vi "Save Notebook Rich Text Box.vi"(6 "Backup?":bool, 7 "Default Notebook File Name (Notebook)":string="Notebook", 8 "Error In":errorcluster, 9 "Dialog (F)":bool, 10 "File Path Control":path, 11 ".NET Refnum in":refnum<k24>) -> (0 "Error Out":errorcluster, 1 "cancelled":bool, 2 "File Path out":path, 3 "Rtf Content":string)   [LabVIEW 2021, in "Notebook.lvlib"]
uses:
  Notebook.lvlib
  System.Windows.Forms
  Rich Text Box/Text Format List.ctl
  GUI/GUI.lvlib
  Files/Files.lvlib
  Rich Text Box/Rich Text Box.lvlib
  Strings/Strings.lvlib
panel:
  # "see the License on the block diagram (Ctrl+E or Window:Show Block Diagram)"
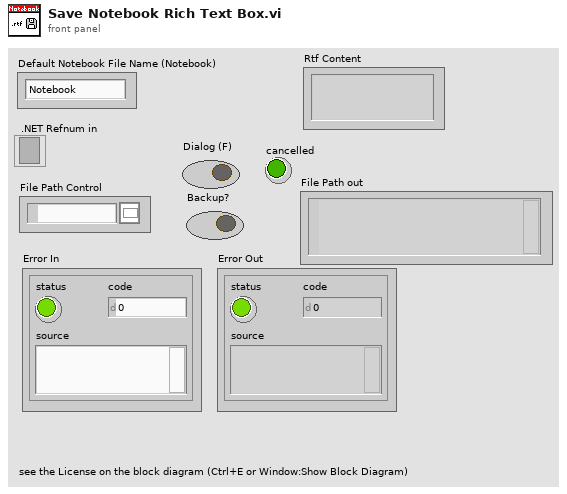
[diagram p1: front panel]
types:
  T1 = typedef "Notebook.lvlib/Text Format List.ctl" = enum16{"Message", "Result", "Error", "Setting", "Verbose", "Warning"}
  T2 = typedef "Rich Text Box.lvlib/Text Formatting.ctl" = cluster{"Font":string, "Text Color":T3, "Background Color":T3, "Style":T4, "Font Size":dbl, "Alignment":T5}
  T3 = typedef "Rich Text Box.lvlib/Text Colors.ctl" = enum16{"Unchanged", "Black", "Blue", "Cyan", "Maroon", "Gray", "Violet", "Green", "Light Green", "Orange", "Yellow", "Magenta", "Red", "White"}
  T4 = typedef "Rich Text Box.lvlib/Text Style.ctl" = enum16{"Regular", "Bold", "Italic", "Underline", "Strikeout"}
  T5 = typedef "Rich Text Box.lvlib/Text Alignment.ctl" = enum16{"Left", "Right", "Center"}
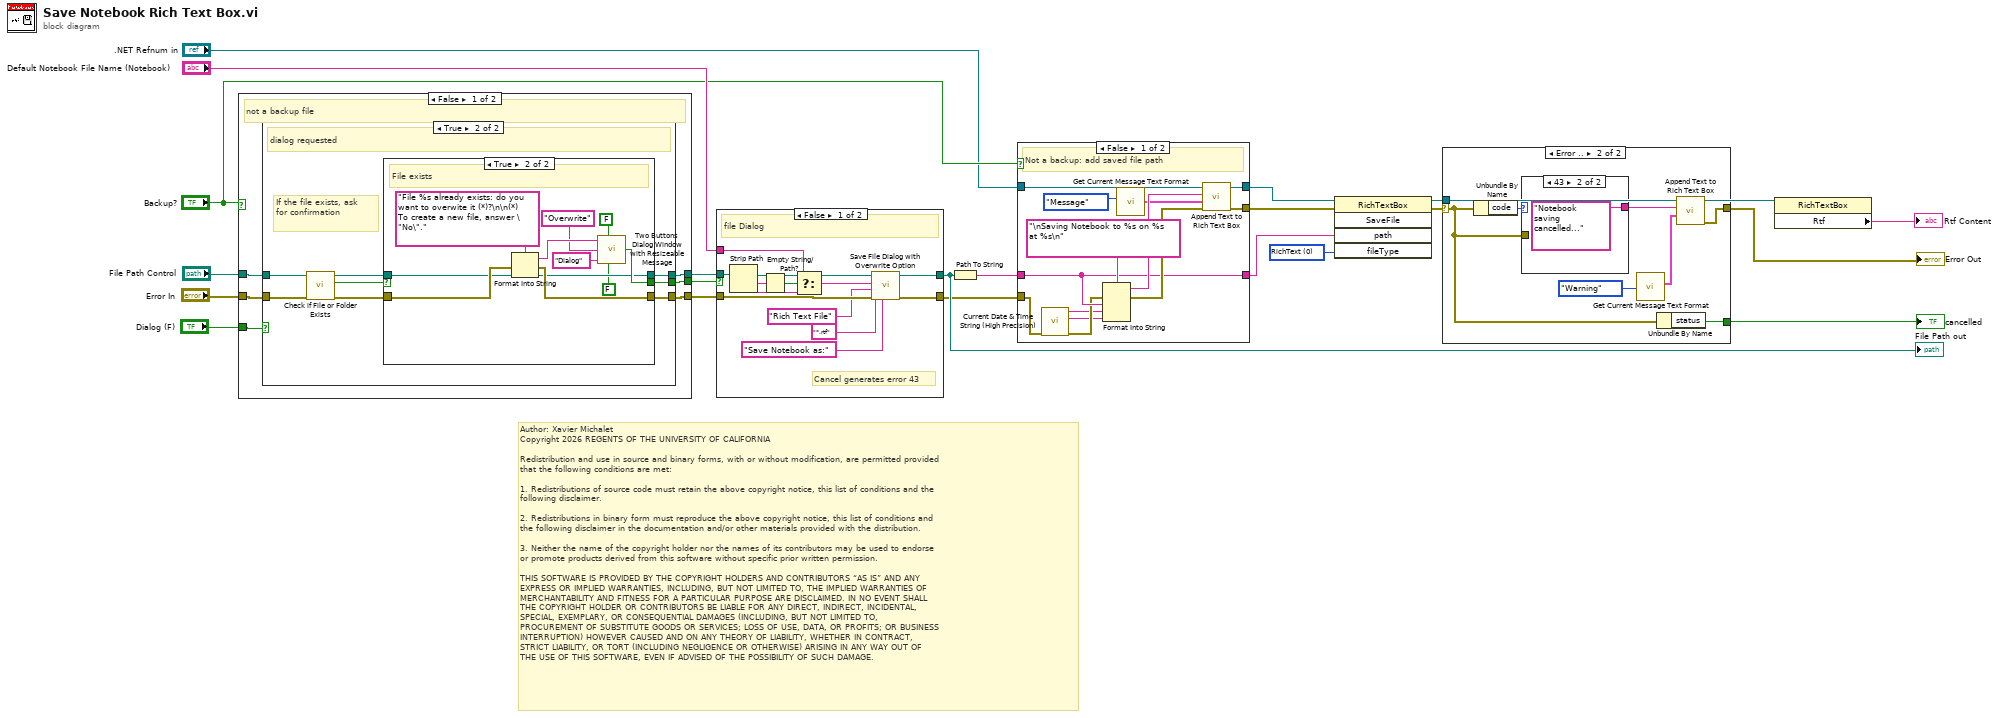
[diagram p0: block diagram]
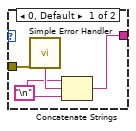
[diagram p4: hidden frame]
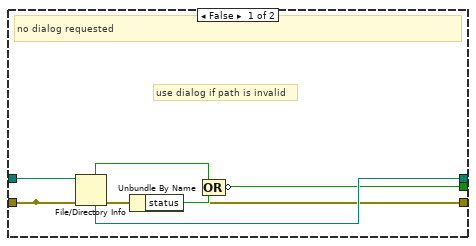
[diagram p6: hidden frame]
diagram:
  w20 = 0 items=["RichText", "PlainText", "RichNoOleObjs", "TextTextOleObjs", "UnicodePlainText"] ("fileType")
  # "Author: Xavier Michalet\nCopyright 2026 REGENTS OF THE UNIVERSITY OF CALIFORNIA\n\nRedistribution and use in source and binary forms, with or without modification, are permitted provided\nthat the following conditions are met:\n\n1. Redistributions of source code must retain the above copyright notice, this list of conditions and the\nfollowing disclaimer.\n\n2. Redistributions in binary form must reproduce the above copyright notice, this list of conditions and\nthe following disclaimer in the documentation and/or other materials provided with the distribution.\n\n3. Neither the name of the copyright holder nor the names of its contributors may be used to endorse \nor promote products derived from this software without specific prior written permission.\n\nTHIS SOFTWARE IS PROVIDED BY THE COPYRIGHT HOLDERS AND CONTRIBUTORS “AS IS” AND ANY \nEXPRESS OR IMPLIED WARRANTIES, INCLUDING, BUT NOT LIMITED TO, THE IMPLIED WARRANTIES OF\nMERCHANTABILITY AND FITNESS FOR A PARTICULAR PURPOSE ARE DISCLAIMED. IN NO EVENT SHALL\nTHE COPYRIGHT HOLDER OR CONTRIBUTORS BE LIABLE FOR ANY DIRECT, INDIRECT, INCIDENTAL, \nSPECIAL, EXEMPLARY, OR CONSEQUENTIAL DAMAGES (INCLUDING, BUT NOT LIMITED TO, \nPROCUREMENT OF SUBSTITUTE GOODS OR SERVICES; LOSS OF USE, DATA, OR PROFITS; OR BUSINESS\nINTERRUPTION) HOWEVER CAUSED AND ON ANY THEORY OF LIABILITY, WHETHER IN CONTRACT, \nSTRICT LIABILITY, OR TORT (INCLUDING NEGLIGENCE OR OTHERWISE) ARISING IN ANY WAY OUT OF\nTHE USE OF THIS SOFTWARE, EVEN IF ADVISED OF THE POSSIBILITY OF SUCH DAMAGE."
  n1 = case shown="False" "Backup?" {
    selector: "Backup?" -> [_ w58]
    tunnel: [w25 w57] -> w19
    tunnel: [w27 w56] -> w18
    tunnel: [w26 w58] -> w17
    tunnel: "Dialog (F)" -> [w22 _]
    tunnel: "File Path Control" -> [w24 w57]
    tunnel: "Error In" -> [w23 w56]
    frame False {
      # "not a backup file"
      n2 = case shown="True" w22 {
        tunnel: [w28 w42] -> w27
        tunnel: [w29 w41] -> w26
        tunnel: [w33 w40] -> w25
        tunnel: w24 -> [w34 w39]
        tunnel: w23 -> [w28 w38]
        frame False {
          # "use dialog if path is invalid"
          # "no dialog requested"
          n3 = File/Directory Info(path=w34, error in=w28) -> (directory=w30:bool, error out=w32:errorcluster, resolved path=w33:path)  [unwired: 4 out]
          n4 = Unbundle By Name(w32) -> ("status"=w31:bool)
          n5 = Compound Arithmetic op=OR(w30, w31) -> (invert w29:bool)
        }
        frame True {
          # "If the file exists, ask for confirmation"
          # "dialog requested"
          n6 = call <vilib>:"Check if File or Folder Exists.vi"("error in (no error)"=w38, "path"=w39) -> ("error out"=w37:errorcluster, "file or folder exists?"=w35:bool, "dup path"=w36:path)  [unwired: 7 in]
          n7 = case shown="True" w35 {
            selector: w35 -> [w43 _]
            tunnel: w37 -> [w44 w53]
            tunnel: [w44 w52] -> w42
            tunnel: [w43 w49] -> w41
            tunnel: w36 -> [w45 w48]
            tunnel: [w45 w48] -> w40
            frame False {
              # "File does not exist"
            }
            frame True {
              # "File exists"
              n8 = Format Into String(format string="File %s already exists: do you want to overwite it (*)?\n\n(*) To create a new file, answer \"No\".", error in=w53, w48) -> (resulting string=w54:string, error out=w52:errorcluster)  [unwired: 1 in]
              n9 = call "Two Buttons Dialog Window with Resizeable Message.vi"("Message"=w54, "Return =  OK (T)"=FALSE, "OK Button Text"="Overwrite" ("T button name (\"OK\")"), "Cancel Button Text"="Dialog" ("F button name (\"Cancel\")"), "ESC =  Cancel (T)"=FALSE) -> ("OK?"=w49:bool)  [unwired: 4 in]
            }
          }
        }
      }
    }
    frame True {
      # "backup: no dialog"
    }
  }
  n10 = case shown="False" w17 {
    tunnel: [w69 w71] -> w21
    tunnel: [w68 w72] -> w8
    tunnel: w19 -> [w67 w71]
    tunnel: w18 -> [w66 w72]
    tunnel: "Default Notebook File Name (Notebook)" -> [w59 _]
    frame False {
      # "Cancel generates error 43"
      # "file Dialog"
      n11 = Strip Path(path=w67) -> (stripped path=w65:path, name=w60:string)
      n12 = Empty String/Path?(string/path=w60) -> (empty?=w62:bool)
      n13 = Select(t=w59, s=w62, f=w60) -> (s? t:f=w61:string)
      n14 = call "Save File Dialog with Overwrite Option.vi"("prompt"="Save Notebook as:", "Default Name"=w61, "error in (no error)"=w66, "pattern label"="Rich Text File", "pattern (all files)"="*.rtf" ("pattern label"), "Starting Folder"=w65) -> ("error out"=w68:errorcluster, "selected path"=w69:path)  [unwired: 2 in, 2 out]
    }
    frame True {
      # "no dialog needed"
    }
  }
  "File Path out" <- w21
  n15 = Path To String(path=w21) -> (string=w4:string)
  n16 = case shown="False" "Backup?" {
    tunnel: ".NET Refnum in" -> [w85 w86]
    tunnel: [w84 w88] -> w12
    tunnel: w8 -> [w79 w88]
    tunnel: w4 -> [w80 w87]
    tunnel: [w80 w87] -> w5
    tunnel: [w75 w86] -> w1
    frame False {
      # "Not a backup: add saved file path"
      n17 = call "Current Date & Time String (High Precision).vi"("Error In"=w79) -> ("Error Out"=w78:errorcluster, "time string"=w76:string, "date string"=w77:string)  [unwired: 7 in, 1 out]
      n18 = Format Into String(format string="\nSaving Notebook to %s on %s at %s\n", error in=w78, w80, w77, w76) -> (resulting string=w82:string, error out=w83:errorcluster)  [unwired: 1 in]
      n19 = call "Get Current Message Text Format.vi"("Text Format"=Text_Format_List."Message") -> ("Message Formatting"=w73:T2)  [unwired: 8 in, 1 out]
      n20 = call "Append Text to Rich Text Box.vi"("error in (no error)"=w83, "Text Formatting"=w73, "String"=w82, ".NET Refnum in"=w85) -> ("Error Out"=w84:errorcluster, ".NET Refnum out"=w75:refnum<k24>)  [unwired: 5 in, 1 out]
    }
    frame True {
      # "backup file"
    }
  }
  n21 = invoke class="RichTextBox" method="SaveFile"(reference=w1, error in=w12, "path"=w5, "fileType"=w20) -> (reference out=w9:refnum<k24>, error out=w11:errorcluster)  [unwired: 1 in, 3 out]
  n22 = case shown="Error .." w11 {
    selector: w11 -> [w89 w91]
    tunnel: [w89 w95] -> w3
    tunnel: [_ w97] -> w10
    tunnel: w9 -> [_ w96]
    frame No Error {
    }
    frame Error {
      n23 = Unbundle By Name(w91) -> ("code"=w93:i32)
      n24 = case shown="43" w93 {
        tunnel: [w99 "Notebook saving cancelled..." ("String")] -> w92
        tunnel: w91 -> [w101 _]
        frame 0, Default {
          w98 = "\n"
          n25 = call <vilib>:"Simple Error Handler.vi"("error in (no error)"=w101) -> ("message"=w100:string)  [unwired: 4 in, 4 out]
          n26 = Concatenate Strings(w98, w100, w98) -> (w99:string)
        }
        frame 43 {
        }
      }
      n27 = call "Get Current Message Text Format.vi"("Text Format"=Text_Format_List."Warning") -> ("Message Formatting"=w94:T2)  [unwired: 8 in, 1 out]
      n28 = Unbundle By Name(w91) -> ("status"=w97:bool)
      n29 = call "Append Text to Rich Text Box.vi"("Text Formatting"=w94, "String"=w92, ".NET Refnum in"=w96) -> ("Error Out"=w95:errorcluster)  [unwired: 6 in, 2 out]
    }
  }
  "Error Out" <- w3
  "cancelled" <- w10
  n30 = property class="RichTextBox"(reference=w9) -> ("Rtf"=→"Rtf Content":string)  [unwired: 1 in, 2 out]
